vi "write report_v2.vi"(0 "fixed filename":string="out.txt", 1 "filename":string, 2 "input":string, 3 "Multiple File?":bool, 4 "file path (use dialog)":path=path "C:/Users/Garnet/Desktop/New folder/LabView Program/RDUW_v2/Independent") -> ()   [LabVIEW 2010]
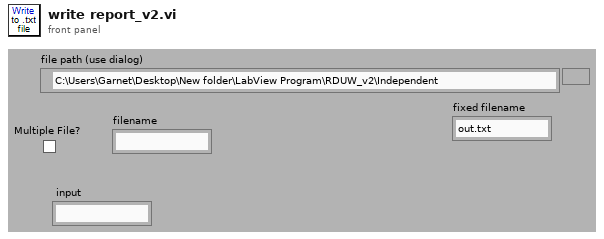
[diagram p1: front panel]
types:
  T1 = enum16{"open", "replace", "create", "open or create", "replace or create", "replace or create with confirmation"}
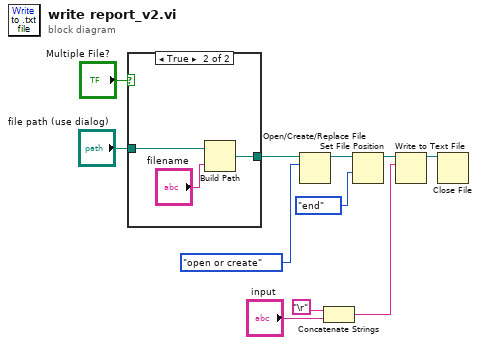
[diagram p0: block diagram]
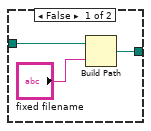
[diagram p2: hidden frame]
diagram:
  n1 = case shown="True" "Multiple File?" {
    tunnel: "file path (use dialog)" -> [w14 w16]
    tunnel: [w12 w17] -> w1
    frame False {
      n2 = Build Path(base path=w14, name or relative path="fixed filename") -> (appended path=w12:path)
    }
    frame True {
      n3 = Build Path(base path=w16, name or relative path="filename") -> (appended path=w17:path)
    }
  }
  n4 = Open/Create/Replace File(file path (use dialog)=w1, operation (0:open)=T1."open or create") -> (refnum out=w11:refnum<file>)  [unwired: 4 in, 2 out]
  n5 = Concatenate Strings("\r", "input") -> (w5:string)
  n6 = Set File Position(refnum=w11, from (0:start)=enum16{"start", "end", "current"}."end") -> (refnum out=w9:refnum<file>)  [unwired: 2 in, 1 out]
  n7 = Write to Text File(file (use dialog)=w9, text=w5) -> (refnum out=w8:refnum<file>)  [unwired: 2 in, 2 out]
  n8 = Close File(refnum=w8) -> ()  [unwired: 1 in, 2 out]
